vi "Get Test Config File Content.vi"(8 "error in (no error)":errorcluster, 11 "Configuration Manager Test in":refnum<class "Configuration Manager Test.lvclass">) -> (0 "error out":errorcluster, 2 "File Content":string, 3 "Configuration Manager Test out":refnum<class "Configuration Manager Test.lvclass">)   [LabVIEW 2020, in "Configuration Manager Test.lvclass"]
uses:
  Configuration Manager Test.lvclass
  Configuration Manager Test.lvclass/Configuration Manager Test.ctl
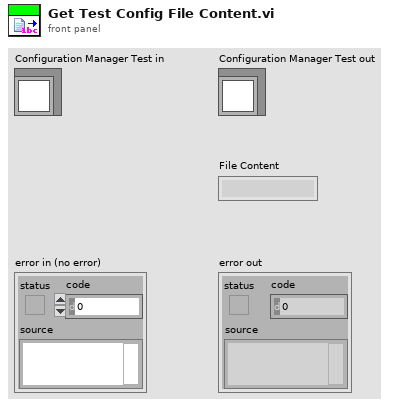
[diagram p1: front panel]
types:
  T1 = enum16{"open", "replace", "create", "open or create", "replace or create", "replace or create with confirmation"}
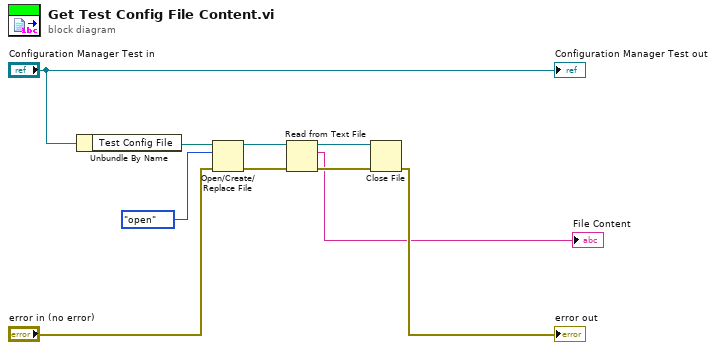
[diagram p0: block diagram]
diagram:
  n1 = Unbundle By Name("Configuration Manager Test in") -> ("Test Config File"=w2:path)
  n2 = Open/Create/Replace File(file path (use dialog)=w2, error in="error in (no error)", operation (0:open)=T1."open") -> (refnum out=w10:refnum<file>, error out=w9:errorcluster)  [unwired: 3 in, 1 out]
  n3 = Read from Text File(file (use dialog)=w10, error in=w9) -> (refnum out=w8:refnum<file>, text=→"File Content":string, error out=w7:errorcluster)  [unwired: 2 in, 1 out]
  n4 = Close File(refnum=w8, error in=w7) -> (error out=→"error out":errorcluster)  [unwired: 1 out]
  "Configuration Manager Test out" <- "Configuration Manager Test in"
